vi "Write Unsigned Integer Configuration.vi"(7 "Type":T1, 8 "error in (no error)":errorcluster, 9 "Value":u64, 10 "Name":string, 11 "database-configuration in":refnum<class "configuration-database.lvclass">) -> (0 "error out":errorcluster, 3 "database-configuration out":refnum<class "configuration-database.lvclass">)   [LabVIEW 2020, in "configuration-database.lvlib" / "configuration-database.lvclass"]
uses:
  configuration-database.lvclass
  <vilib>/Utility/Data Type/Type Definitions/Data Type.ctl
  configuration-database.lvclass/configuration-database.ctl
  9ea4760c-a3af-4ef5-b9d4-988a507bb96c.vi
  <vilib>/Utility/error.llb/Error Cluster From Error Code.vi
  IConfigDBQueries/IConfigurationDatabaseQueries.lvclass
  externals/database-interface/IDatabase/IDatabase/IDatabase.lvclass
  <vilib>/Utility/Data Type/NI_Data Type.lvlib
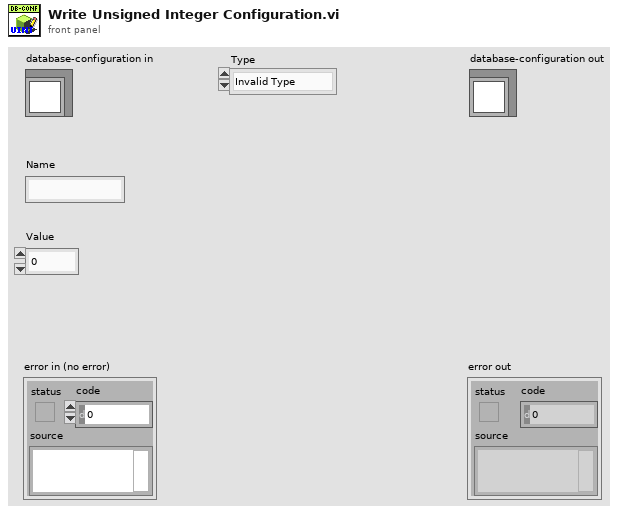
[diagram p1: front panel]
types:
  T1 = typedef "NI_Data Type.lvlib/Data Type.ctl" = enum8{"Invalid Type", "Void", "I8", "I16", "I32", "I64", "U8", "U16", "U32", "U64", "Single Float", "Double Float", "Extended Float", "Single Complex", "Double Complex", "Extended Complex", "Enum U8", "Enum U16", "Enum U32", "Enum U64", "Single Float With Unit", "Double Float With Unit", "Extended Float With Unit", "Single Complex with Unit", "Double Complex with Unit", "Extended Complex with Unit", "Boolean", "String", "Path", "Picture", "Tag", "Array", "Cluster", "Variant", "LV Variant", "Waveform", "Timestamp", "Digital Waveform", "Digital Data", "ExpressData", "Refnum", "External Data", "VI", "Poly VI", "LabVIEW Class Instance", "Fixed Point", "Set Collection", "Map Collection"}
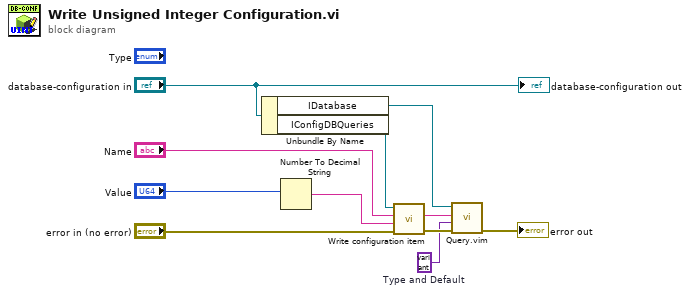
[diagram p0: block diagram]
diagram:
  w1 = variant  # Type and Default
  n1 = Unbundle By Name("database-configuration in") -> ("IDatabase"=w3:refnum<class "IDatabase.lvclass">, "IConfigDBQueries"=w9:refnum<class "IConfigurationDatabaseQueries.lvclass">)
  n2 = Number To Decimal String(number="Value") -> (decimal integer string=w8:string)  [unwired: 1 in]
  n3 = call-dynamic "Write configuration item.vi"("error in (no error)"="error in (no error)", "Value"=w8, "Name in"="Name", "IConfigDBQueries in"=w9) -> ("error out"=w10:errorcluster, "Query"=w11:string)  [unwired: 6 in]
  n4 = call "Query.vim"("error in (no error)"=w10, "Type and Default"=w1, "Query string"=w11, "IDatabase in"=w3) -> ("error out"=→"error out":errorcluster)  [unwired: 5 in, 2 out]
  "database-configuration out" <- "database-configuration in"
